vi "Read Sweep Control.json.vi"(8 "error in (no error)":errorcluster, 10 "file (use dialog)":path, 11 "SweepControl in":refnum<class "Sweep Control.lvclass">) -> (0 "error out":errorcluster, 2 "data":T1={"Experiment"=enum."Lockin_DelayLine", "Repeat Experiment"=0, "Scan control"=[], "Scan parameters"=[]} {"Scan parameters"."Rate" format="%.2f"; "Scan parameters"."Step" format="%#_6p"; "Scan parameters"."End" format="%#_6p"; "Scan parameters"."Start" format="%#_6p"; "Repeat Experiment" min=1}, 3 "SweepControl out":refnum<class "Sweep Control.lvclass">)   [LabVIEW 2019, in "Sweep Control.lvclass"]
uses:
  Sweep Control.lvclass
  Typedefs/Sweep Control JSON--Cluster.ctl
  Typedefs/Enum - Experiments.ctl
  Typedefs/ScanControl.ctl
  Typedefs/Cluster - ScanControl.ctl
  Typedefs/Enum - Priority.ctl
  Typedefs/Enum - Action.ctl
  Typedefs/ScanParamters.ctl
  Typedefs/Cluster - ScanParamters.ctl
  6bb5f8be-f1e2-427f-a6d8-5173d26fd901.vi
  <vilib>/JDP Science/JSONtext/JSON text to Variant.vi
  <vilib>/JDP Science/JSONtext/LVClass Serializer/JSONtext LVClass Serializer.lvclass
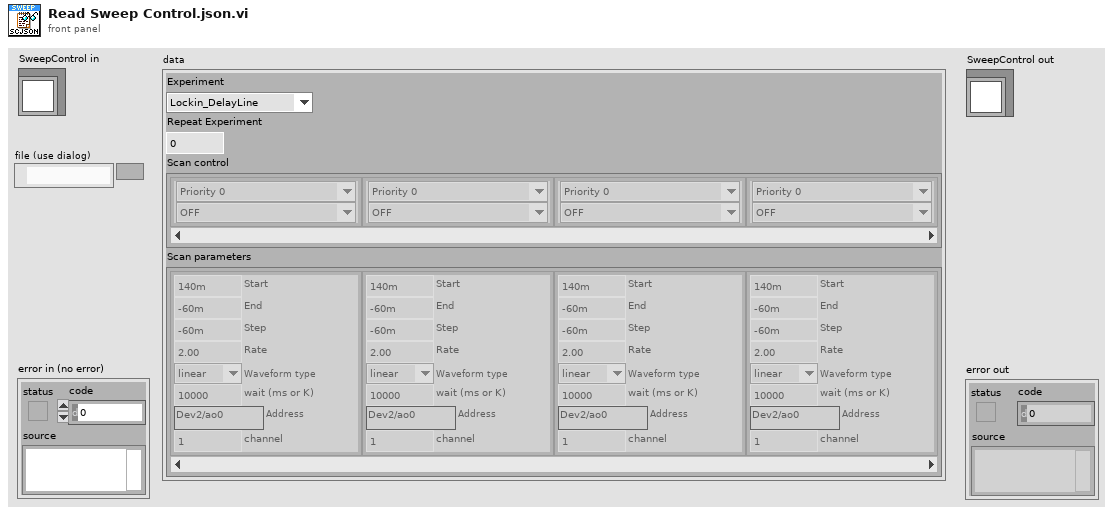
[diagram p1: front panel]
types:
  T1 = typedef "Sweep Control.lvclass/Sweep Control JSON--Cluster.ctl" = cluster{"Experiment":T2, "Repeat Experiment":i32, "Scan control":T3, "Scan parameters":T7}
  T2 = typedef "Sweep Control.lvclass/Enum - Experiments.ctl" = enum16{"Lockin_time", "Lockin_sweep", "Lockin_DelayLine"}
  T3 = typedef "Sweep Control.lvclass/ScanControl.ctl" = T4[]
  T4 = typedef "Sweep Control.lvclass/Cluster - ScanControl.ctl" = cluster{"Priority":T5, "Scan name":T6}
  T5 = typedef "Sweep Control.lvclass/Enum - Priority.ctl" = enum16{"Priority 0", "Priority 1", "Priority 2", "Priority 3", "Priority 4", "Priority 5"}
  T6 = typedef "Sweep Control.lvclass/Enum - Action.ctl" = enum16{"OFF", "time", "Lockin Amplitude", "Lockin Frequency", "Lockin Bias", "Delay", "Strain", "DAQ Bias", "Magnet Field", "Temperature", "MW f1", "MW f2", "MW Amplitude1", "MW Amplitude2"}
  T7 = typedef "Sweep Control.lvclass/ScanParamters.ctl" = T8[]
  T8 = typedef "Sweep Control.lvclass/Cluster - ScanParamters.ctl" = cluster{"Start":dbl, "End":dbl, "Step":dbl, "Rate":dbl, "Waveform type":enum16{"linear", "triangle", "power"}, "wait (ms or K)":dbl, "Address":string, "channel":i32}
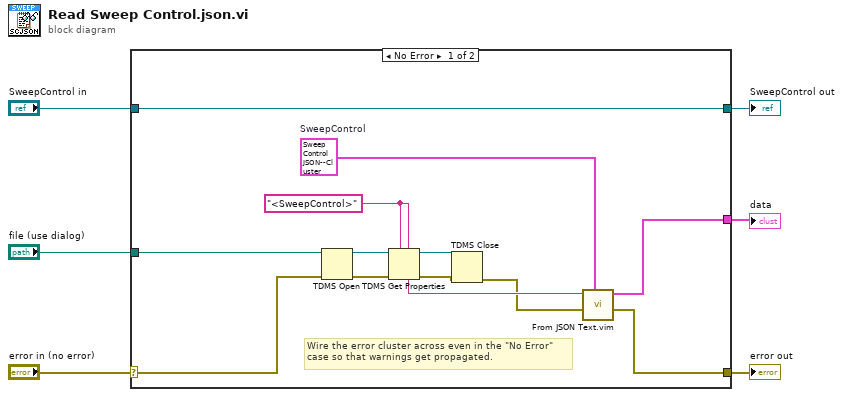
[diagram p0: block diagram]
diagram:
  n1 = case shown="No Error" "error in (no error)" {
    selector: "error in (no error)" -> [w14 w21]
    tunnel: [w8 w21] -> w5
    tunnel: [w19 w20] -> w3
    tunnel: "SweepControl in" -> [w19 w20]
    tunnel: "file (use dialog)" -> [w13 _]
    tunnel: [w9 _] -> w1
    frame No Error {
      w18 = "<SweepControl>" ("group name")
      w10 = T1 {"Experiment"=enum."Lockin_DelayLine", "Repeat Experiment"=0, "Scan control"=[], "Scan parameters"=[]}  # SweepControl
      # "Wire the error cluster across even in the \"No Error\"\ncase so that warnings get propagated."
      n2 = TDMS Open(8:w14, 11:w13) -> (0:w12:errorcluster, 3:w17:refnum<k34>)  [unwired: 5 in]
      n3 = TDMS Get Properties(5:w18, 7:w18, 8:w12, 11:w17) -> (0:w11:errorcluster, 3:w16:refnum<k34>, 4:w15:string)  [unwired: 2 in, 3 out]
      n4 = TDMS Close(8:w11, 11:w16) -> (0:w7:errorcluster)  [unwired: 1 out]
      n5 = call "From JSON Text.vim"("Data Type and Default Value"=w10, "error in (no error)"=w7, "JSON"=w15) -> ("error out"=w8:errorcluster, "Data out"=w9:T1)  [unwired: 7 in]
    }
    frame Error {
    }
  }
  "error out" <- w5
  "SweepControl out" <- w3
  "data" <- w1
